vi "CRYSet Constant to TipStrip.vi"(8 "Work in":u16(slide), 11 "Constant":dbl format="%#.5p") -> (1 "Tip Out":string)   [LabVIEW 2013]
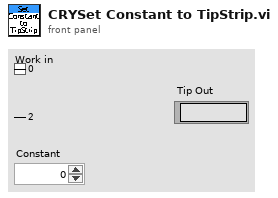
[diagram p1: front panel]
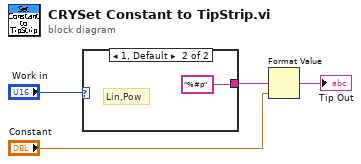
[diagram p0: block diagram]
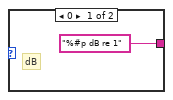
[diagram p2: hidden frame]
diagram:
  n1 = case shown="1, Default" "Work in" {
    tunnel: ["%#p dB re 1" ("format string") "%#p" ("format string")] -> w3
    frame 0 {
      # "dB"
    }
    frame 1, Default {
      # "Lin,Pow"
    }
  }
  n2 = Format Value(format string=w3, value (0)="Constant") -> (output string=→"Tip Out":string)  [unwired: 1 in]
